vi "Ref_StsP.vi"(0 "Status Ch 1":refnum<vi>, 1 "Status Ch 2":refnum<vi>, 2 "Status Ch 3":refnum<vi>, 3 "Status Ch 4":refnum<vi>, 4 "Status Ch 5":refnum<vi>, 5 "Status Ch 6":refnum<vi>, 6 "Status Ch 7":refnum<vi>, 7 "Status Ch 8":refnum<vi>, 8 "Status Ch 9":refnum<vi>, 9 "Status Ch 10":refnum<vi>, 10 "Status Ch 11":refnum<vi>, 11 "Status Ch 12":refnum<vi>, 14 "Init_F":bool=TRUE) -> (16 "Status Ch11 out":refnum<vi>, 17 "Status Ch12 out":refnum<vi>, 18 "Status Ch9 out":refnum<vi>, 19 "Status Ch10 out":refnum<vi>, 20 "Status Ch1 out":refnum<vi>, 21 "Status Ch2 out":refnum<vi>, 22 "Status Ch3 out":refnum<vi>, 23 "Status Ch4 out":refnum<vi>, 24 "Status Ch5 out":refnum<vi>, 25 "Status Ch6 out":refnum<vi>, 26 "Status Ch7 out":refnum<vi>, 27 "Status Ch8 out":refnum<vi>)   [LabVIEW 2017]
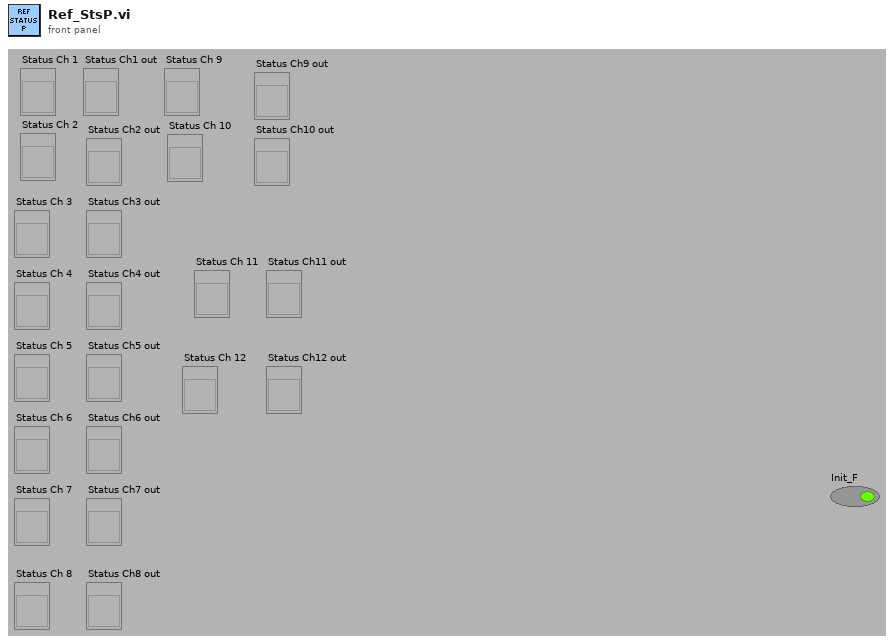
[diagram p1: front panel]
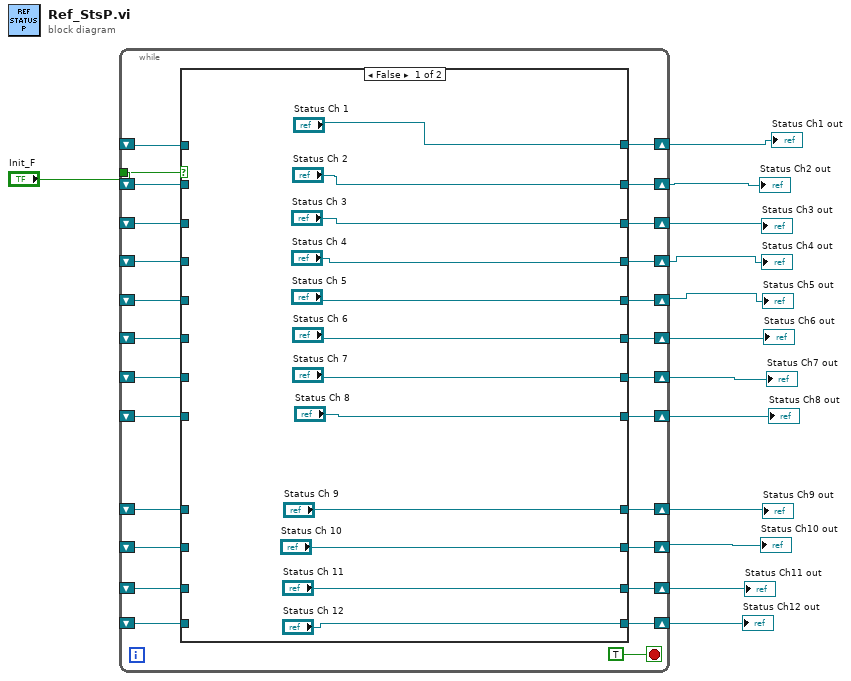
[diagram p0: block diagram]
diagram:
  n1 = while {
    shift-right: [w38] -> w12
    shift-left: _ -> [w37]
    tunnel: "Init_F" -> [w36]
    shift-right: [w35] -> w5
    shift-left: _ -> [w28]
    shift-right: [w34] -> w6
    shift-left: _ -> [w27]
    shift-right: [w33] -> w7
    shift-left: _ -> [w22]
    shift-right: [w32] -> w8
    shift-left: _ -> [w26]
    shift-right: [w31] -> w9
    shift-left: _ -> [w25]
    shift-right: [w30] -> w10
    shift-left: _ -> [w24]
    shift-right: [w29] -> w11
    shift-left: _ -> [w23]
    shift-right: [w21] -> w3
    shift-left: _ -> [w19]
    shift-right: [w20] -> w4
    shift-left: _ -> [w18]
    shift-right: [w17] -> w2
    shift-left: _ -> [w15]
    shift-right: [w16] -> w1
    shift-left: _ -> [w14]
    stop <- TRUE stop-if-true
    n2 = case shown="False" w36 {
      tunnel: ["Status Ch 1" w63] -> w38
      tunnel: w37 -> [_ w63]
      tunnel: ["Status Ch 2" w56] -> w35
      tunnel: ["Status Ch 3" w57] -> w34
      tunnel: ["Status Ch 4" w58] -> w33
      tunnel: ["Status Ch 5" w59] -> w32
      tunnel: ["Status Ch 6" w60] -> w31
      tunnel: ["Status Ch 7" w61] -> w30
      tunnel: ["Status Ch 8" w62] -> w29
      tunnel: w28 -> [_ w56]
      tunnel: w27 -> [_ w57]
      tunnel: w26 -> [_ w59]
      tunnel: w25 -> [_ w60]
      tunnel: w24 -> [_ w61]
      tunnel: w23 -> [_ w62]
      tunnel: w22 -> [_ w58]
      tunnel: ["Status Ch 9" w55] -> w21
      tunnel: ["Status Ch 10" w54] -> w20
      tunnel: w19 -> [_ w55]
      tunnel: w18 -> [_ w54]
      tunnel: ["Status Ch 11" w53] -> w17
      tunnel: ["Status Ch 12" w52] -> w16
      tunnel: w15 -> [_ w53]
      tunnel: w14 -> [_ w52]
      frame False {
      }
      frame True {
      }
    }
  }
  "Status Ch1 out" <- w12
  "Status Ch2 out" <- w5
  "Status Ch3 out" <- w6
  "Status Ch4 out" <- w7
  "Status Ch5 out" <- w8
  "Status Ch6 out" <- w9
  "Status Ch7 out" <- w10
  "Status Ch8 out" <- w11
  "Status Ch9 out" <- w3
  "Status Ch10 out" <- w4
  "Status Ch11 out" <- w2
  "Status Ch12 out" <- w1
